vi "Status Get Register.vi"(8 "error in (no error)":errorcluster {"code" format="%.0x"}, 9 "Register (Standard Event)":i32(ring)=11 items=["Standard Event"=11, "Standard Event Enable"=12, "Status Byte"=13, "Service Request Enable"=10, "Operation Condition"=0, "Operation Event"=2, "Operation Negative Transition"=3, "Operation Positive Transition"=4, "Questionable Condition"=5, "Questionable Event"=7, "Questionable Negative Transition"=8, "Questionable Positive Transition"=9, "Questionable Enable"=6, "Operation Enable"=1, "Operation Instrument Condition"=14, "Operation Instrument Enable"=15, "Operation Instrument Event"=16, "Operation Instrument Negative Transition"=17, "Operation Instrument Positive Transition"=18, "Questionable Calibration Condition"=19, "Questionable Calibration Enable"=20, "Questionable Calibration Event"=21, "Questionable Calibration Extended Failure Condition"=22, "Questionable Calibration Extended Failure Enable"=23, "Questionable Calibration Extended Failure Event"=24, "Questionable Calibration Extended Failure Negative Transition"=25, "Questionable Calibration Extended Failure Positive Transition"=26, "Questionable Calibration Extended Needed Condition"=27, "Questionable Calibration Extended Needed Enable"=28, "Questionable Calibration Extended Needed Event"=29, "Questionable Calibration Extended Needed Negative Transition"=30, "Questionable Calibration Extended Needed Positive Transition"=31, "Questionable Calibration Negative Transition"=32, "Questionable Calibration Positive Transition"=33, "Questionable Calibration Skipped Condition"=34, "Questionable Calibration Skipped Enable"=35, "Questionable Calibration Skipped Event"=36, "Questionable Calibration Skipped Negative Transition"=37, "Questionable Calibration Skipped Positive Transition"=38, "Questionable Frequency Condition"=39, "Questionable Frequency Enable"=40, "Questionable Frequency Event"=41, "Questionable Frequency Negative Transition"=42, "Questionable Frequency Positive Transition"=43, "Questionable Integrity Condition"=44, "Questionable Integrity Enable"=45, "Questionable Integrity Event"=46, "Questionable Integrity Negative Transition"=47, "Questionable Integrity Positive Transition"=48, "Questionable Integrity Signal Condition"=49, "Questionable Integrity Signal Enable"=50, "Questionable Integrity Signal Event"=51, "Questionable Integrity Signal Negative Transition"=52, "Questionable Integrity Signal Positive Transition"=53, "Questionable Integrity Un Calibrated Condition"=54, "Questionable Integrity Un Calibrated Enable"=55, "Questionable Integrity Un Calibrated Event"=56, "Questionable Integrity Un Calibrated Negative Transition"=57, "Questionable Integrity Un Calibrated Positive Transition"=58, "Questionable Power Condition"=59, "Questionable Power Enable"=60, "Questionable Power Event"=61, "Questionable Power Negative Transition"=62, "Questionable Power Positive Transition"=63, "Questionable Temperature Condition"=64, "Questionable Temperature Enable"=65, "Questionable Temperature Event"=66, "Questionable Temperature Negative Transition"=67, "Questionable Temperature Positive Transition"=68], 11 "instrument handle":refnum<k15>) -> (0 "error out":errorcluster {"code" format="%.0x"}, 2 "Val":i16, 3 "instrument handle out":refnum<k15>)   [LabVIEW 2021, in "Keysight XSAnVMA.lvlib"]
doc: "Gets the specified instrument status register. Reading an Event register clears it. Other registers are unaffected."
uses:
  <instrlib>/Keysight XSAnVMA/Keysight XSAnVMA.lvlib
  KtXSAnVMA_64.dll
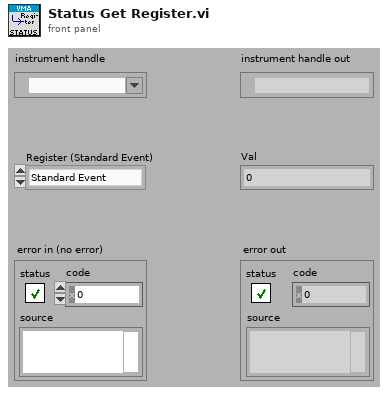
[diagram p1: front panel]
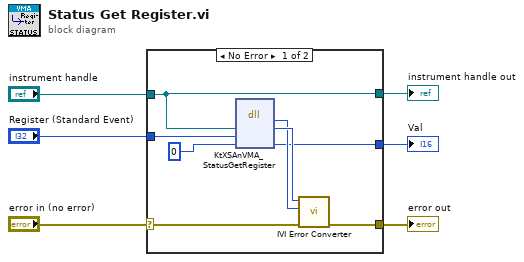
[diagram p0: block diagram]
diagram:
  n1 = case shown="No Error" "error in (no error)" {
    selector: "error in (no error)" -> [w12 w16]
    tunnel: [w11 w16] -> w6
    tunnel: "instrument handle" -> [w7 w15]
    tunnel: "Register (Standard Event)" -> [w10 _]
    tunnel: [w8 _] -> w2
    tunnel: [w7 w15] -> w1
    frame No Error {
      n2 = dll-call lib="KtXSAnVMA**.dll" fn="KtXSAnVMA_StatusGetRegister"("Vi"=w7, "Register"=w10, "Val"=i16 0) -> (w13:i32, "Vi"=w14:u32, "Val"=w8:i16)  [unwired: 4 in, 2 out]
      n3 = call <instrlib>:"IVI Error Converter.vi"("error in (no error)"=w12, "IVI error code (0)"=w13, "instrument handle"=w14) -> ("error out"=w11:errorcluster)  [unwired: 7 in, 1 out]
    }
    frame Error {
    }
  }
  "error out" <- w6
  "instrument handle out" <- w1
  "Val" <- w2
